vi "SaveWriteSetupFile.vi"(8 "Error In":errorcluster, 10 "Setup":T1={"Slots"=[], "Memory"=[], "Scan List"="", "Trigger"={"Arm"={"Source"=enum."Hold", "Count"=1, "Infinite?"=FALSE}, "Scan"={"Source"=enum."Hold", "Count"=0, "Infinite?"=FALSE, "Delay (sec)"=0.0, "Interval (sec)"=0.0}, "Channel"={"Source"=enum."Hold", "Count"=0, "Infinite?"=FALSE, "Auto Count?"=FALSE, "Delay (sec)"=0.0, "Interval (sec)"=0.0}}} {"Trigger"."Arm"."Count" min=1 max=99999 step=1}, 11 "Save File":path) -> (0 "Error Out":errorcluster)   [LabVIEW 2012]
uses:
  Setup.ctl
  SlotConfiguration.ctl
  BankConfiguration.ctl
  TriggerConfiguration.ctl
  TriggerArmConfiguration.ctl
  driver/Public/Controls/ArmSource.ctl
  TriggerScanConfiguration.ctl
  driver/Public/Controls/ScanSource.ctl
  TriggerChannelConfiguration.ctl
  driver/Public/Controls/TriggerSource.ctl
  <vilib>/xml/Close Reference(Node).vi
  <vilib>/xml/NI_XML.lvlib
  <resource>/objmgr/DOMUserDefRef.rc
  libs/LV-Utilities/LV-Utilities.lvlib
  driver/Keithley-7001.lvlib
panel:
  out "XML":string
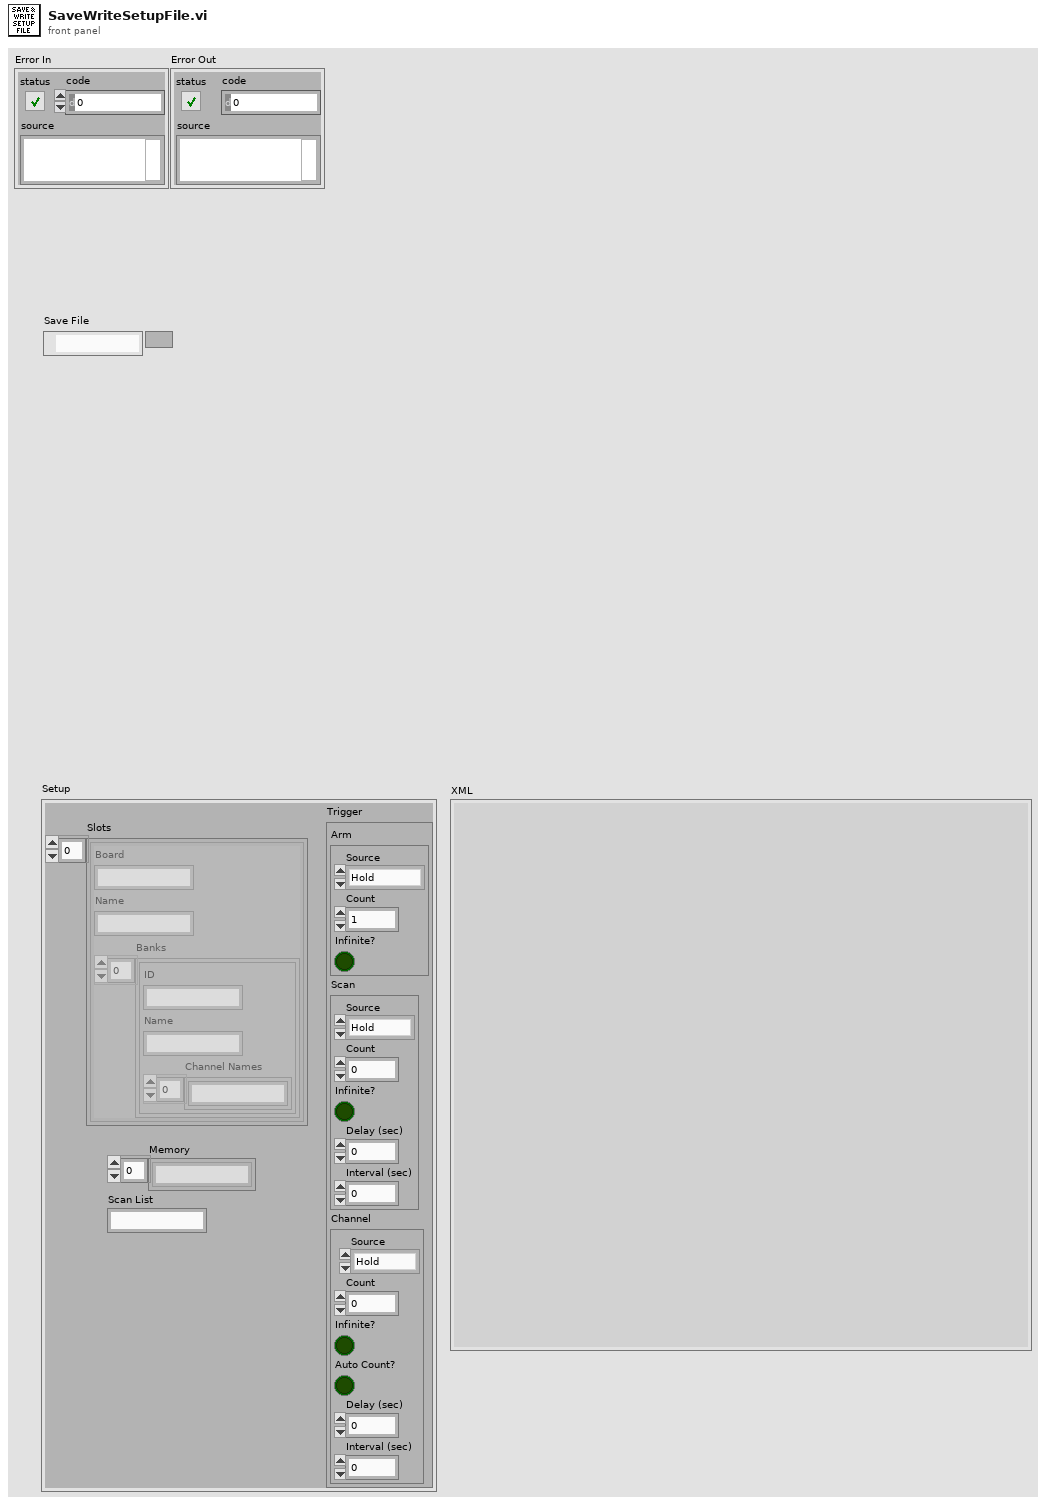
[diagram p1: front panel]
types:
  T1 = typedef "Setup.ctl" = cluster{"Slots":T2[], "Memory":string[], "Scan List":string, "Trigger":T4}
  T2 = typedef "SlotConfiguration.ctl" = cluster{"Board":string, "Name":string, "Banks":T3[]}
  T3 = typedef "BankConfiguration.ctl" = cluster{"ID":string, "Name":string, "Channel Names":string[]}
  T4 = typedef "TriggerConfiguration.ctl" = cluster{"Arm":T5, "Scan":T7, "Channel":T9}
  T5 = typedef "TriggerArmConfiguration.ctl" = cluster{"Source":T6, "Count":u32, "Infinite?":bool}
  T6 = typedef "Keithley-7001.lvlib/ArmSource.ctl" = enum16{"Hold", "Immediate", "Manual", "Bus", "TLink", "External"}
  T7 = typedef "TriggerScanConfiguration.ctl" = cluster{"Source":T8, "Count":u32, "Infinite?":bool, "Delay (sec)":dbl, "Interval (sec)":dbl}
  T8 = typedef "Keithley-7001.lvlib/ScanSource.ctl" = enum16{"Hold", "Immediate", "Timer", "Manual", "Bus", "TLink", "External"}
  T9 = typedef "TriggerChannelConfiguration.ctl" = cluster{"Source":T10, "Count":u32, "Infinite?":bool, "Auto Count?":bool, "Delay (sec)":dbl, "Interval (sec)":dbl}
  T10 = typedef "Keithley-7001.lvlib/TriggerSource.ctl" = enum16{"Hold", "Immediate", "Manual", "Bus", "TLink", "External", "Timer"}
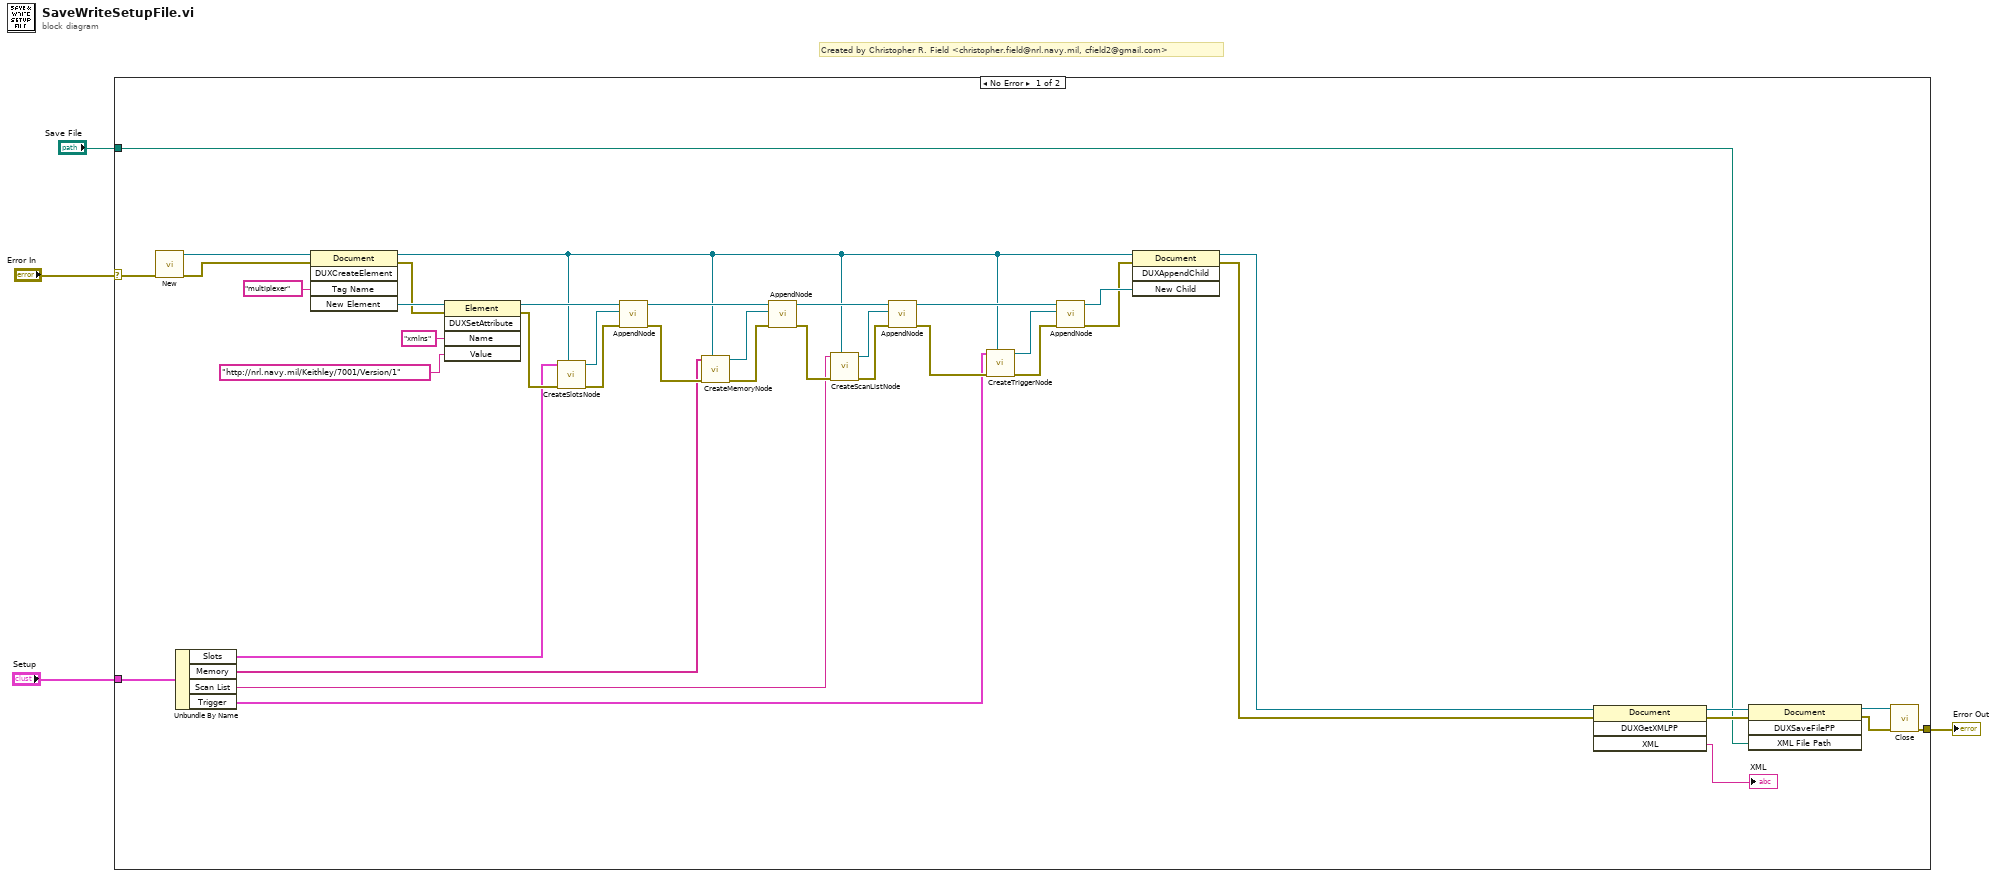
[diagram p0: block diagram]
diagram:
  # "Created by Christopher R. Field <christopher.field@nrl.navy.mil, cfield2@gmail.com>"
  n1 = case shown="No Error" "Error In" {
    selector: "Error In" -> [w45 w46]
    tunnel: "Save File" -> [w38 _]
    tunnel: [w39 w46] -> w2
    tunnel: "Setup" -> [w13 _]
    frame No Error {
      n2 = call <vilib>:"New.vi"("error in (no error)"=w45) -> ("error out"=w31:errorcluster, "DOM document out"=w32:refnum<k20>)  [unwired: 7 in]
      n3 = Unbundle By Name(w13) -> ("Slots"=w5:T2[], "Memory"=w12:string[], "Scan List"=w11:string, "Trigger"=w10:T4)
      n4 = invoke class="Document" method="DUXCreateElement"(reference=w32, error in=w31, "Tag Name"="multiplexer") -> (reference out=w9:refnum<k20>, error out=w35:errorcluster, "New Element"=w36:refnum<k20>)  [unwired: 2 in, 2 out]
      n5 = invoke class="Element" method="DUXSetAttribute"(reference=w36, error in=w35, "Name"="xmlns", "Value"="http://nrl.navy.mil/Keithley/7001/Version/1") -> (reference out=w30:refnum<k20>, error out=w6:errorcluster)  [unwired: 1 in, 3 out]
      n6 = call "CreateSlotsNode.vi"("DOM Document"=w9, "Error In"=w6, "Slots"=w5) -> ("Error Out"=w8:errorcluster, "Slots Node"=w7:refnum<k20>)  [unwired: 7 in]
      n7 = call "AppendNode.vi"("Error In"=w8, "Child Node"=w7, "Parent Node In"=w30) -> ("Error Out"=w29:errorcluster, "Parent Node Out"=w28:refnum<k20>)  [unwired: 7 in]
      n8 = call "CreateMemoryNode.vi"("DOM Document"=w9, "Error In"=w29, "Memory"=w12) -> ("Error Out"=w26:errorcluster, "Memory Node"=w27:refnum<k20>)  [unwired: 7 in]
      n9 = call "AppendNode.vi"("Error In"=w26, "Child Node"=w27, "Parent Node In"=w28) -> ("Error Out"=w25:errorcluster, "Parent Node Out"=w24:refnum<k20>)  [unwired: 7 in]
      n10 = call "CreateScanListNode.vi"("DOM Document"=w9, "Error In"=w25, "Scan List"=w11) -> ("Error Out"=w22:errorcluster, "Scan List Node"=w23:refnum<k20>)  [unwired: 7 in]
      n11 = call "AppendNode.vi"("Error In"=w22, "Child Node"=w23, "Parent Node In"=w24) -> ("Error Out"=w21:errorcluster, "Parent Node Out"=w20:refnum<k20>)  [unwired: 7 in]
      n12 = call "CreateTriggerNode.vi"("DOM Document"=w9, "Error In"=w21, "Trigger Configuration"=w10) -> ("Error Out"=w18:errorcluster, "Trigger Node"=w19:refnum<k20>)  [unwired: 7 in]
      n13 = call "AppendNode.vi"("Error In"=w18, "Child Node"=w19, "Parent Node In"=w20) -> ("Error Out"=w16:errorcluster, "Parent Node Out"=w17:refnum<k20>)  [unwired: 7 in]
      n14 = invoke class="Document" method="DUXAppendChild"(reference=w9, error in=w16, "New Child"=w17) -> (reference out=w14:refnum<k20>, error out=w15:errorcluster)  [unwired: 1 in, 2 out]
      n15 = invoke class="Document" method="DUXGetXMLPP"(reference=w14, error in=w15) -> (reference out=w44:refnum<k20>, error out=w43:errorcluster, "XML"=→"XML":string)  [unwired: 2 in, 1 out]
      n16 = invoke class="Document" method="DUXSaveFilePP"(reference=w44, error in=w43, "XML File Path"=w38) -> (reference out=w42:refnum<k20>, error out=w41:errorcluster)  [unwired: 1 in, 2 out]
      n17 = call-poly <vilib>:"Close.vi"("error in (no error)"=w41, "node"=w42) -> ("error out"=w39:errorcluster)  [unwired: 7 in]
    }
    frame Error {
    }
  }
  "Error Out" <- w2
